vi "oa_OneShot VS AutoRestart.vi"(11 "error in (no error)":errorcluster, 12 "averaging parameters":T2={"averaging mode"=enum."No averaging", "weighting mode"=enum."Exponential", "number of averages"=10, "linear mode"=enum."One shot"} {"number of averages" min=1 step=1}, 13 "averaging done":bool) -> (14 "processing control out":T1(ring), 15 "error out":errorcluster)   [LabVIEW 2017, in "SoundVib_Resampling.lvlib"]
uses:
  <vilib>/addons/Sound and Vibration/Order Analysis/Resample Order Tracking/SoundVib_Resampling.lvlib
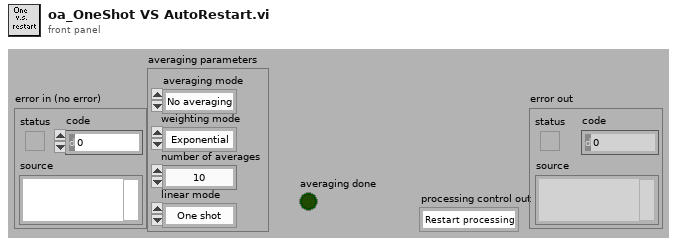
[diagram p1: front panel]
types:
  T1 = enum16{"Restart processing", "Continue processing", "Skip processing"}
  T2 = cluster{"averaging mode":enum16{"No averaging", "Vector averaging", "RMS averaging", "Peak hold"}, "weighting mode":enum16{"Linear", "Exponential"}, "number of averages":u32, "linear mode":enum16{"One shot", "Auto restart"}}
  T3 = enum16{"No averaging", "Vector averaging", "RMS averaging", "Peak hold"}
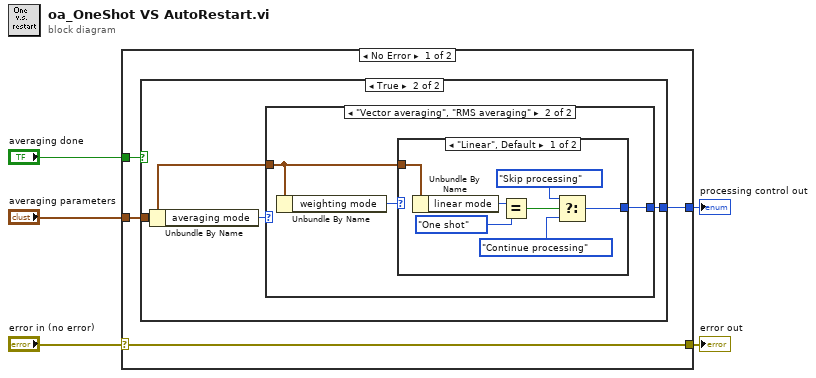
[diagram p0: block diagram]
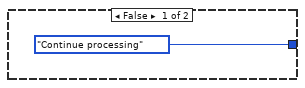
[diagram p2: hidden frame]
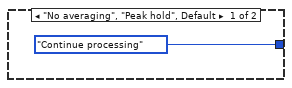
[diagram p3: hidden frame]
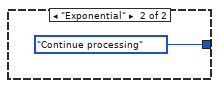
[diagram p4: hidden frame]
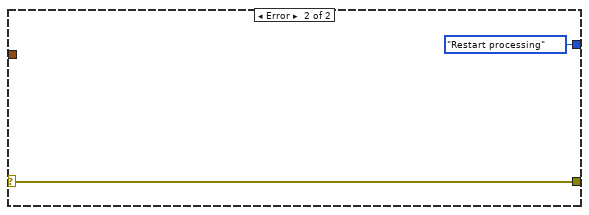
[diagram p5: hidden frame]
diagram:
  n1 = case shown="No Error" "error in (no error)" {
    selector: "error in (no error)" -> [w9 w27]
    tunnel: [w9 w27] -> w4
    tunnel: "averaging done" -> [w8 _]
    tunnel: [w7 T1."Restart processing"] -> w2
    tunnel: "averaging parameters" -> [w6 _]
    frame No Error {
      n2 = case shown="True" w8 {
        tunnel: [T1."Continue processing" ("processing control out") w11] -> w7
        tunnel: w6 -> [_ w13]
        frame False {
        }
        frame True {
          n3 = Unbundle By Name(w13) -> ("averaging mode"=w12:T3)
          n4 = case shown="\"Vector averaging\", \"RMS averaging\"" w12 {
            tunnel: w13 -> [_ w17]
            tunnel: [T1."Continue processing" ("processing control") w16] -> w11
            frame "No averaging", "Peak hold", Default {
            }
            frame "Vector averaging", "RMS averaging" {
              n5 = Unbundle By Name(w17) -> ("weighting mode"=w15:enum16{"Linear", "Exponential"})
              n6 = case shown="\"Linear\", Default" w15 {
                tunnel: w17 -> [w24 _]
                tunnel: [w18 T1."Continue processing" ("processing control")] -> w16
                frame "Linear", Default {
                  n7 = Unbundle By Name(w24) -> ("linear mode"=w23:enum16{"One shot", "Auto restart"})
                  n8 = Equal?(x=w23, y=enum16{"One shot", "Auto restart"}."One shot") -> (x = y?=w21:bool)
                  n9 = Select(t=T1."Skip processing" ("processing control"), s=w21, f=T1."Continue processing" ("processing control")) -> (s? t:f=w18:T1)
                }
                frame "Exponential" {
                }
              }
            }
          }
        }
      }
    }
    frame Error {
    }
  }
  "processing control out" <- w2
  "error out" <- w4
